vi "RT_RW_ADCs_W_DAC.vi"() -> ()   [LabVIEW 2018]
uses:
  <vilib>/FPGAPlugInAG/myRIO-1900/niLvFpga_Open_myRIO-1900.vi
  <vilib>/rvi/interface/common/dynamic/niFpgaDynamicAddResources.vi
  <vilib>/Utility/error.llb/Error Cluster From Error Code.vi
  <vilib>/rvi/errors/niLvFpgaAdjustHostInterfaceError.vi
  <vilib>/rvi/interface/nirviOpenFPGA/nirviOpenFPGA.xnode
  FPGA Bitfiles/ASPE2019amplifie_FPGATarget_fpgaW&RADCsW3DAC_bDaL8r7O+ms.lvbitx
  <vilib>/rvi/interface/nirviReadWriteControl/nirviReadWriteControl.xnode
  NiFpgaLv.dll
  <vilib>/rvi/interface/Simulation/niFpgaSimulationCallBeginRW.vi
panel:
  out "CH 4":dbl(graph)=-2.3028213070479264
  out "CH 3":dbl(graph)=-2.30221096479851
  out "CH 2":dbl(graph)=-2.301905793673802
  in  "ADC 1 write":bool[](array[boolean])=[FALSE, FALSE, FALSE, FALSE, FALSE, TRUE, FALSE, FALSE, FALSE, FALSE, FALSE, FALSE, FALSE, FALSE, FALSE, FALSE]
  in  "ADC 4 write":bool[](array[boolean])=[FALSE, FALSE, TRUE, TRUE, FALSE, TRUE, FALSE, FALSE, FALSE, FALSE, FALSE, FALSE, FALSE, FALSE, FALSE, FALSE]
  in  "ADC 3 write":bool[](array[boolean])=[FALSE, FALSE, TRUE, FALSE, FALSE, TRUE, FALSE, FALSE, FALSE, FALSE, FALSE, FALSE, FALSE, FALSE, FALSE, FALSE]
  in  "ADC 2 write":bool[](array[boolean])=[FALSE, FALSE, FALSE, TRUE, FALSE, TRUE, FALSE, FALSE, FALSE, FALSE, FALSE, FALSE, FALSE, FALSE, FALSE, FALSE]
  out "loop rate (kHz)":dbl=52.43735814798003
  in  "DAC (V)":dbl
  in  "Stop Button":bool
  out "CH1 (V)":dbl(graph)=-2.30221096479851
  # "All channels are configured to read +/-10 V range in differential mode"
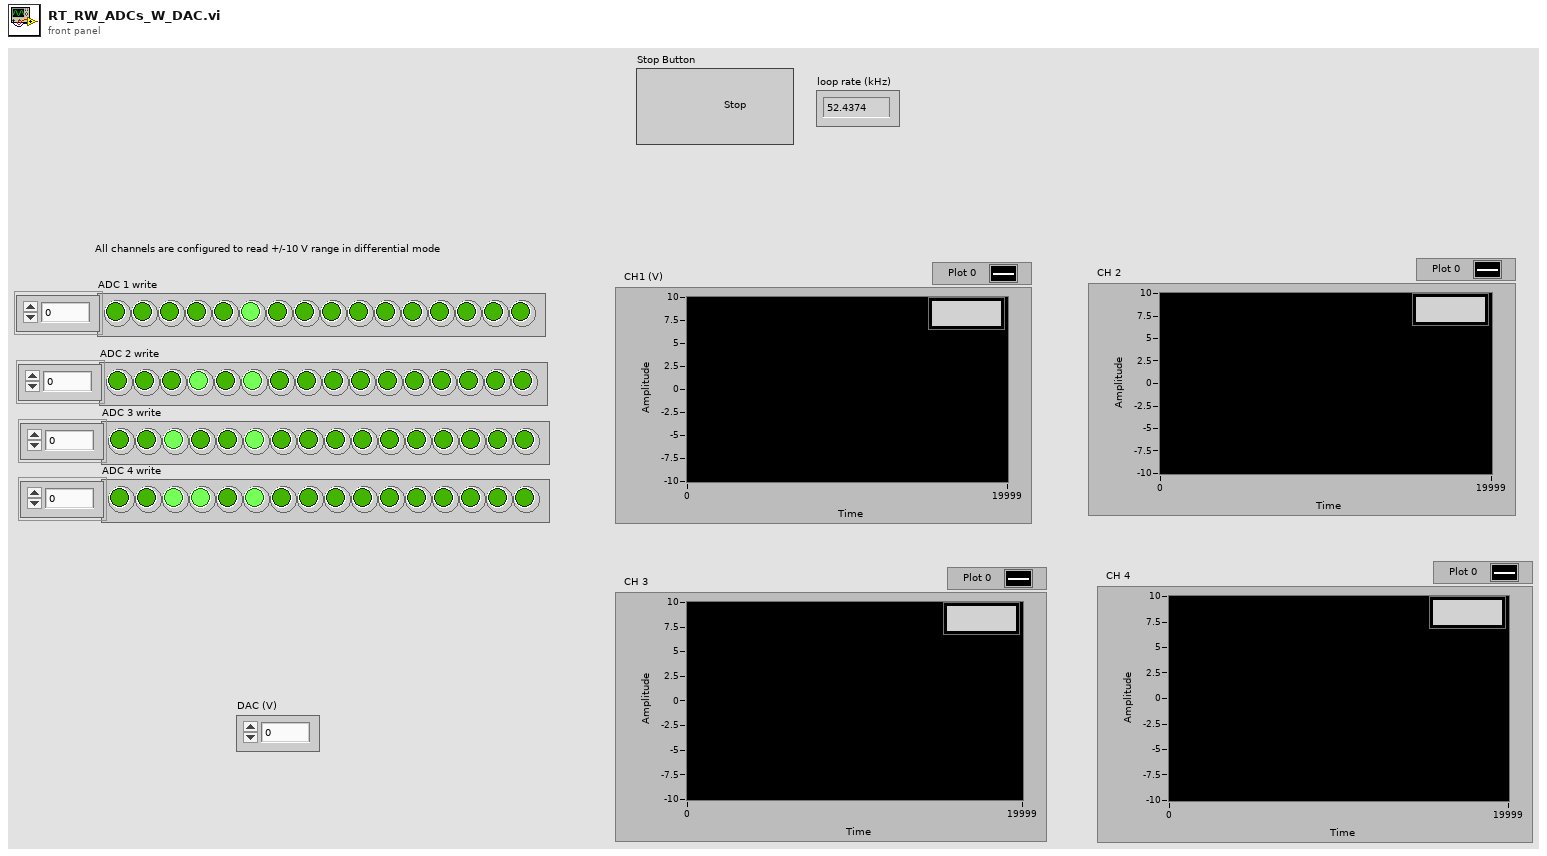
[diagram p1: front panel]
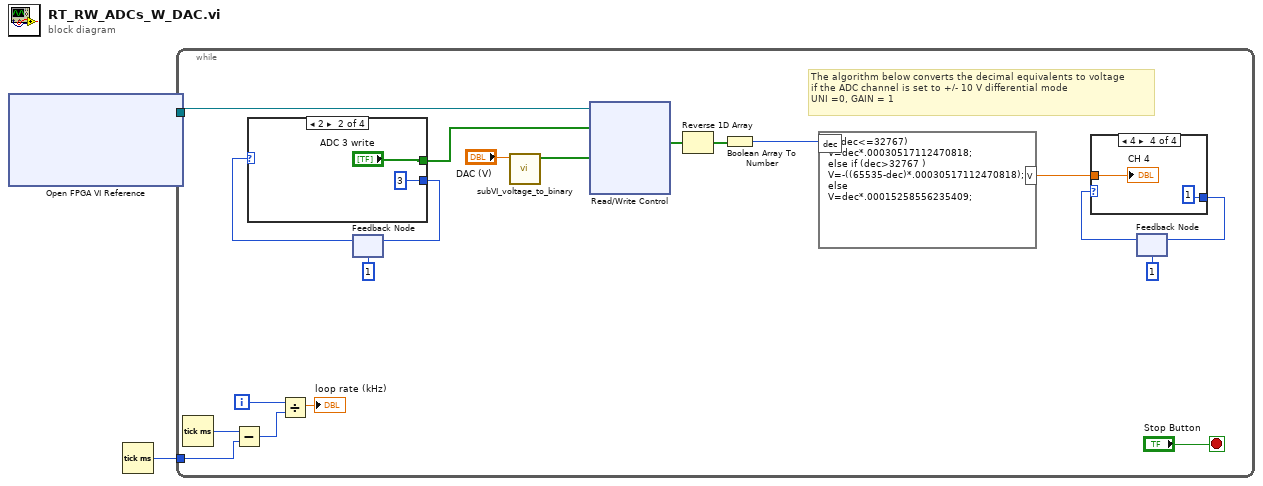
[diagram p0: block diagram]
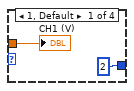
[diagram p2: hidden frame]
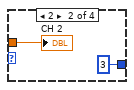
[diagram p3: hidden frame]
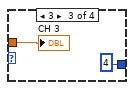
[diagram p4: hidden frame]
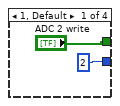
[diagram p5: hidden frame]
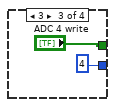
[diagram p6: hidden frame]
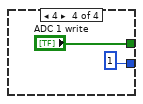
[diagram p7: hidden frame]
diagram:
  n1 = xnode "Open FPGA VI Reference"() -> ("FPGA VI Reference Out"=w2:refnum<k20>)  [unwired: 2 in, 1 out]
  n2 = Tick Count (ms)() -> (millisecond timer value=w1:u32)
  n3 = while {
    tunnel: w2 -> [w22]
    tunnel: w1 -> [w17]
    i -> [w16]
    stop <- "Stop Button" stop-if-true
    # "The algorithm below converts the decimal equivalents to voltage\nif the ADC channel is set to +/- 10 V differential mode\nUNI =0, GAIN = 1"
    n4 = Tick Count (ms)() -> (millisecond timer value=w18:u32)
    n5 = Subtract(x=w18, y=w17) -> (x-y=w15:u32)
    n6 = Divide(x=w16, y=w15) -> (x/y=→"loop rate (kHz)":dbl)
    n7 = feedback #1(u8 1) -> (w11:u8)
    n8 = case shown="2" w11 {
      tunnel: [u8 2 u8 3 u8 4 u8 1] -> w10
      tunnel: ["ADC 2 write" "ADC 3 write" "ADC 4 write" "ADC 1 write"] -> w9
      frame 1, Default {
      }
      frame 2 {
      }
      frame 3 {
      }
      frame 4 {
      }
    }
    n9 = feedback-in #1(w10) -> ()
    n10 = call "subVI_voltage_to_binary.vi"("voltage"="DAC (V)") -> ("binary"=w3:bool[])  [unwired: 10 in]
    n11 = xnode "Read/Write Control"("FPGA VI Reference In"=w22, "ADC write"=w9, "DAC 1 write"=w3) -> ("ADC read"=w19:bool[])  [unwired: 3 in, 2 out]
    n12 = Reverse 1D Array(array=w19) -> (reversed array=w20:bool[])
    n13 = Boolean Array To Number(Boolean array=w20) -> (number=w13:u16)
    n14 = formula code="if (dec<=32767)\nV=dec*.00030517112470818;\nelse if (dec>32767 )\nV=-((65535-dec)*.00030517112470818);\nelse\nV=dec*.00015258556235409;"("dec"=w13) -> ("V"=w6:dbl)
    n15 = feedback #2(u8 1) -> (w8:u8)
    n16 = case shown="4" w8 {
      tunnel: [u8 2 u8 3 u8 4 u8 1] -> w7
      tunnel: w6 -> [w23 w25 w27 w29]
      frame 1, Default {
        "CH1 (V)" <- w23
      }
      frame 2 {
        "CH 2" <- w25
      }
      frame 3 {
        "CH 3" <- w27
      }
      frame 4 {
        "CH 4" <- w29
      }
    }
    n17 = feedback-in #2(w7) -> ()
  }
